vi "ArrayOfSinglesToByteArray.vi"(5 "Values":sgl[](array[numeric])) -> (2 "unsigned byte array":u8[](array[numeric]))   [LabVIEW 2017, in "ServerComm.lvlib"]
uses:
  <vilib>/addons/InsightCM/Devices/Shared/Common/ServerComm/ServerComm.lvlib
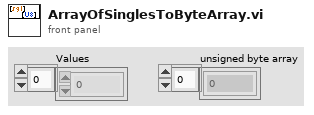
[diagram p1: front panel]
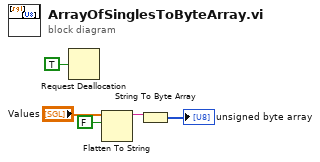
[diagram p0: block diagram]
diagram:
  n1 = Request Deallocation(TRUE ("flag")) -> ()
  n2 = Flatten To String(anything="Values", prepend array or string size? (T)=FALSE) -> (data string=w4:string)  [unwired: 2 in, 2 out]
  n3 = String To Byte Array(string=w4) -> (unsigned byte array=→"unsigned byte array":u8[])
